vi "SV FRF State Manager.vi"(0 "FRF State":T10 {"spectrum info"."x-axis units" items=["Time (s)"=0, "Frequency-CB (Hz)"=1, "Frequency-CPB (Hz)"=1248, "Frequency-Arbitrary (Hz)"=2357, "Quefrency (s)"=2, "Revolutions (rev)"=3, "Order"=4, "Speed (RPM)"=11, "Speed (rad/s)"=21, "Index"=65535]; "spectrum info"."weighting filter" items=["Linear", "A-weighting", "B-weighting", "C-weighting", "ITU-R 468-4", "Dolby", "CCITT", "C-message", "Wb", "Wc", "Wd", "We", "Wf", "Wh", "Wj", "Wk", "Wm", "AES17 20 kHz lowpass", "AES17 40 kHz lowpass", "AES17 20 kHz highpass", "AES17 40 kHz highpass"]; "spectrum info"."dB reference [EU]" format="%.2f"; "spectrum info"."engineering units" items=["custom..."=0, "V"=1, "A"=21, "C"=30, "pC"=31, "s"=32, "-"=29, "Pa"=2, "N"=20, "g"=3, "m/s^2"=4, "m/s"=5, "m"=6, "mm/s"=12, "mm"=13, "micron/s"=14, "micron"=15, "in/s^2"=7, "in/s"=8, "in"=9, "mil/s"=10, "mil"=11, "rad/s^2"=16, "rad/s"=17, "rad"=18, "deg/s^2"=26, "deg/s"=27, "deg"=28, "RPM"=22, "cycle/s^2"=23, "Hz"=24, "cycle"=25, "strain"=19]; "spectrum info"."spectral info"."window" items=["None "=0, "Hanning"=1, "Hamming"=2, "Blackman-Harris"=3, "Exact Blackman"=4, "Blackman"=5, "Flat Top"=6, "4 Term B-Harris "=7, "7 Term B-Harris"=8, "Low Sidelobe"=9, "Force - Exponential"=10, "Gaussian"=62]; "Data"."coherence"."coherence" format="%.2f"; "Data"."coherence"."df" format="%.2f"; "Data"."coherence"."f0" format="%.2f"; "Data"."phase"."phase" format="%.2f"; "Data"."phase"."df" format="%.2f"; "Data"."phase"."f0" format="%.2f"; "Data"."magnitude"."magnitude" format="%.2p"; "Data"."magnitude"."df" format="%.2p"; "Data"."magnitude"."f0" format="%.2p"; "IDentifiers"."response node"."active node" format="%04.0f"; "IDentifiers"."reference node"."active node" format="%04.0f"}, 2 "Node IDentifiers":T8={"reference node"={"active node"=0, "coordinate"="+Y"}, "response node"={"active node"=0, "coordinate"="+Y"}} {"response node"."active node" format="%04.0f"; "reference node"."active node" format="%04.0f"}, 3 "FRF to add":T9 {"coherence"."coherence" format="%.2f"; "coherence"."df" format="%.2f"; "coherence"."f0" format="%.2f"; "phase"."phase" format="%.2f"; "phase"."df" format="%.2f"; "phase"."f0" format="%.2f"; "magnitude"."magnitude" format="%.2p"; "magnitude"."df" format="%.2p"; "magnitude"."f0" format="%.2p"}, 4 "spectrum info":T1={"channel name"="", "description"="", "x-axis units"=0, "spectral info"={"spectrum type"=enum."Power [Magnitude^2]", "linear/dB"=enum."linear", "window"=0, "window size"=0, "FFT size"=0}, "engineering units"=0, "custom label"="", "dB reference [EU]"=0.0, "peak units"=enum."rms", "weighting filter"=0, "spectral density?"=FALSE, "unit label"="", "spectrum skewed?"=FALSE, "complimentary spectrum units"=enum."none"} {"x-axis units" items=["Time (s)"=0, "Frequency-CB (Hz)"=1, "Frequency-CPB (Hz)"=1248, "Frequency-Arbitrary (Hz)"=2357, "Quefrency (s)"=2, "Revolutions (rev)"=3, "Order"=4, "Speed (RPM)"=11, "Speed (rad/s)"=21, "Index"=65535]; "weighting filter" items=["Linear", "A-weighting", "B-weighting", "C-weighting", "ITU-R 468-4", "Dolby", "CCITT", "C-message", "Wb", "Wc", "Wd", "We", "Wf", "Wh", "Wj", "Wk", "Wm", "AES17 20 kHz lowpass", "AES17 40 kHz lowpass", "AES17 20 kHz highpass", "AES17 40 kHz highpass"]; "dB reference [EU]" format="%.2f"; "engineering units" items=["custom..."=0, "V"=1, "A"=21, "C"=30, "pC"=31, "s"=32, "-"=29, "Pa"=2, "N"=20, "g"=3, "m/s^2"=4, "m/s"=5, "m"=6, "mm/s"=12, "mm"=13, "micron/s"=14, "micron"=15, "in/s^2"=7, "in/s"=8, "in"=9, "mil/s"=10, "mil"=11, "rad/s^2"=16, "rad/s"=17, "rad"=18, "deg/s^2"=26, "deg/s"=27, "deg"=28, "RPM"=22, "cycle/s^2"=23, "Hz"=24, "cycle"=25, "strain"=19]; "spectral info"."window" items=["None "=0, "Hanning"=1, "Hamming"=2, "Blackman-Harris"=3, "Exact Blackman"=4, "Blackman"=5, "Flat Top"=6, "4 Term B-Harris "=7, "7 Term B-Harris"=8, "Low Sidelobe"=9, "Force - Exponential"=10, "Gaussian"=62]}, 6 "action":u16(ring)=3 items=["Initialize to Empty", "Update State", "Delete from State", "Get Identifiers", "Get State"]) -> (12 "state changed":bool, 14 "FRF State out":T10 {"spectrum info"."x-axis units" items=["Time (s)"=0, "Frequency-CB (Hz)"=1, "Frequency-CPB (Hz)"=1248, "Frequency-Arbitrary (Hz)"=2357, "Quefrency (s)"=2, "Revolutions (rev)"=3, "Order"=4, "Speed (RPM)"=11, "Speed (rad/s)"=21, "Index"=65535]; "spectrum info"."weighting filter" items=["Linear", "A-weighting", "B-weighting", "C-weighting", "ITU-R 468-4", "Dolby", "CCITT", "C-message", "Wb", "Wc", "Wd", "We", "Wf", "Wh", "Wj", "Wk", "Wm", "AES17 20 kHz lowpass", "AES17 40 kHz lowpass", "AES17 20 kHz highpass", "AES17 40 kHz highpass"]; "spectrum info"."dB reference [EU]" format="%.2f"; "spectrum info"."engineering units" items=["custom..."=0, "V"=1, "A"=21, "C"=30, "pC"=31, "s"=32, "-"=29, "Pa"=2, "N"=20, "g"=3, "m/s^2"=4, "m/s"=5, "m"=6, "mm/s"=12, "mm"=13, "micron/s"=14, "micron"=15, "in/s^2"=7, "in/s"=8, "in"=9, "mil/s"=10, "mil"=11, "rad/s^2"=16, "rad/s"=17, "rad"=18, "deg/s^2"=26, "deg/s"=27, "deg"=28, "RPM"=22, "cycle/s^2"=23, "Hz"=24, "cycle"=25, "strain"=19]; "spectrum info"."spectral info"."window" items=["None "=0, "Hanning"=1, "Hamming"=2, "Blackman-Harris"=3, "Exact Blackman"=4, "Blackman"=5, "Flat Top"=6, "4 Term B-Harris "=7, "7 Term B-Harris"=8, "Low Sidelobe"=9, "Force - Exponential"=10, "Gaussian"=62]; "Data"."coherence"."coherence" format="%.2f"; "Data"."coherence"."df" format="%.2f"; "Data"."coherence"."f0" format="%.2f"; "Data"."phase"."phase" format="%.2f"; "Data"."phase"."df" format="%.2f"; "Data"."phase"."f0" format="%.2f"; "Data"."magnitude"."magnitude" format="%.2p"; "Data"."magnitude"."df" format="%.2p"; "Data"."magnitude"."f0" format="%.2p"; "IDentifiers"."response node"."active node" format="%04.0f"; "IDentifiers"."reference node"."active node" format="%04.0f"}, 16 "IDentifiers":T7(array[cluster]) {"response node"."active node" format="%04.0f"; "reference node"."active node" format="%04.0f"}, 17 "FRF requested":T9 {"coherence"."coherence" format="%.2f"; "coherence"."df" format="%.2f"; "coherence"."f0" format="%.2f"; "phase"."phase" format="%.2f"; "phase"."df" format="%.2f"; "phase"."f0" format="%.2f"; "magnitude"."magnitude" format="%.2p"; "magnitude"."df" format="%.2p"; "magnitude"."f0" format="%.2p"}, 18 "spectrum info":T1={"channel name"="", "description"="", "x-axis units"=0, "spectral info"={"spectrum type"=enum."Power [Magnitude^2]", "linear/dB"=enum."linear", "window"=0, "window size"=0, "FFT size"=0}, "engineering units"=0, "custom label"="", "dB reference [EU]"=0.0, "peak units"=enum."rms", "weighting filter"=0, "spectral density?"=FALSE, "unit label"="", "spectrum skewed?"=FALSE, "complimentary spectrum units"=enum."none"} {"x-axis units" items=["Time (s)"=0, "Frequency-CB (Hz)"=1, "Frequency-CPB (Hz)"=1248, "Frequency-Arbitrary (Hz)"=2357, "Quefrency (s)"=2, "Revolutions (rev)"=3, "Order"=4, "Speed (RPM)"=11, "Speed (rad/s)"=21, "Index"=65535]; "weighting filter" items=["Linear", "A-weighting", "B-weighting", "C-weighting", "ITU-R 468-4", "Dolby", "CCITT", "C-message", "Wb", "Wc", "Wd", "We", "Wf", "Wh", "Wj", "Wk", "Wm", "AES17 20 kHz lowpass", "AES17 40 kHz lowpass", "AES17 20 kHz highpass", "AES17 40 kHz highpass"]; "dB reference [EU]" format="%.2f"; "engineering units" items=["custom..."=0, "V"=1, "A"=21, "C"=30, "pC"=31, "s"=32, "-"=29, "Pa"=2, "N"=20, "g"=3, "m/s^2"=4, "m/s"=5, "m"=6, "mm/s"=12, "mm"=13, "micron/s"=14, "micron"=15, "in/s^2"=7, "in/s"=8, "in"=9, "mil/s"=10, "mil"=11, "rad/s^2"=16, "rad/s"=17, "rad"=18, "deg/s^2"=26, "deg/s"=27, "deg"=28, "RPM"=22, "cycle/s^2"=23, "Hz"=24, "cycle"=25, "strain"=19]; "spectral info"."window" items=["None "=0, "Hanning"=1, "Hamming"=2, "Blackman-Harris"=3, "Exact Blackman"=4, "Blackman"=5, "Flat Top"=6, "4 Term B-Harris "=7, "7 Term B-Harris"=8, "Low Sidelobe"=9, "Force - Exponential"=10, "Gaussian"=62]})   [LabVIEW 2017]
uses:
  <vilib>/addons/_NISVFA/_Shared subVIs/Controls/svc_Spectrum Info.ctl
  <vilib>/addons/_NISVFA/_Shared subVIs/Controls/svc_X-Axis Units.ctl
  <vilib>/addons/_NISVFA/_Shared subVIs/Controls/svc_Spectrum Type.ctl
  <vilib>/addons/_NISVFA/_Shared subVIs/Controls/svc_Engineering Units Text Ring.ctl
  <vilib>/addons/_NISVFA/_Shared subVIs/Controls/svc_Weighting Filter Text Ring.ctl
  <vilib>/addons/_NISVFA/_Shared subVIs/Controls/svc_Complimentary Spectrum Units.ctl
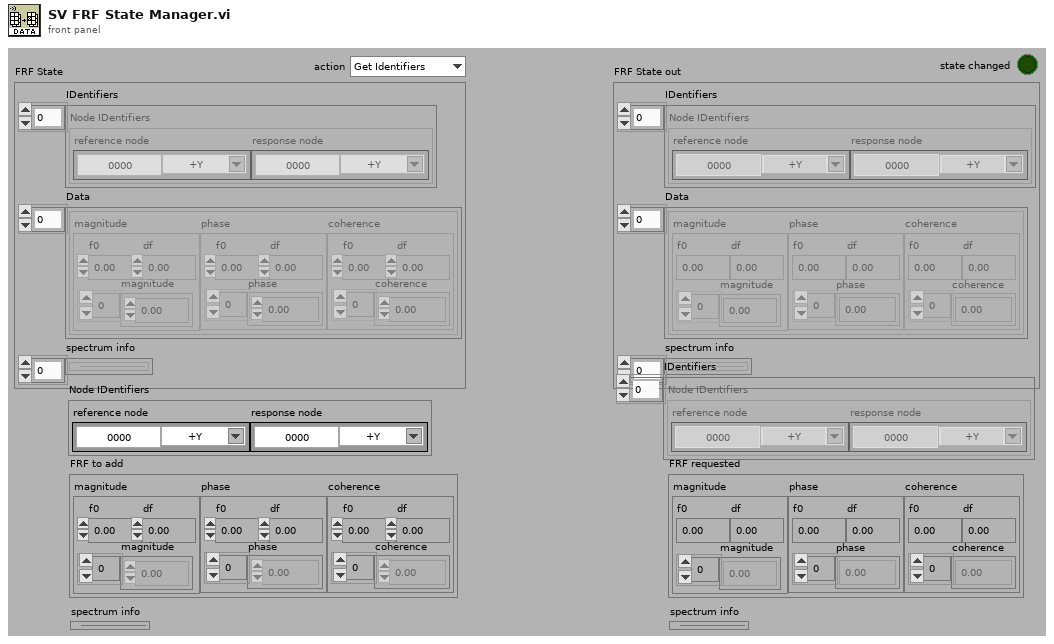
[diagram p1: front panel]
types:
  T1 = typedef "svc_Spectrum Info.ctl" = cluster{"channel name":string, "description":string, "x-axis units":T2, "spectral info":cluster{"spectrum type":T3, "linear/dB":enum16{"linear", "dB"}, "window":u16, "window size":i32, "FFT size":i32}, "engineering units":T4, "custom label":string, "dB reference [EU]":dbl, "peak units":enum16{"rms", "peak", "peak-peak"}, "weighting filter":T5, "spectral density?":bool, "unit label":string, "spectrum skewed?":bool, "complimentary spectrum units":T6}
  T2 = typedef "svc_X-Axis Units.ctl" = u16
  T3 = typedef "svc_Spectrum Type.ctl" = enum16{"FFT Spectrum [complex]", "Amplitude [Magnitude]", "Power [Magnitude^2]", "Cross Spectrum [complex]", "Frequency Response [Complex]"}
  T4 = typedef "svc_Engineering Units Text Ring.ctl" = u16
  T5 = typedef "svc_Weighting Filter Text Ring.ctl" = u16
  T6 = typedef "svc_Complimentary Spectrum Units.ctl" = enum16{"none", "radians", "degrees", "cycles", "imaginary"}
  T7 = cluster{"reference node":cluster{"active node":i32, "coordinate":string}, "response node":cluster{"active node":i32, "coordinate":string}}[]
  T8 = cluster{"reference node":cluster{"active node":i32, "coordinate":string}, "response node":cluster{"active node":i32, "coordinate":string}}
  T9 = cluster{"magnitude":cluster{"f0":dbl, "df":dbl, "magnitude":dbl[]}, "phase":cluster{"f0":dbl, "df":dbl, "phase":dbl[]}, "coherence":cluster{"f0":dbl, "df":dbl, "coherence":dbl[]}}
  T10 = cluster{"IDentifiers":cluster{"reference node":cluster{"active node":i32, "coordinate":string}, "response node":cluster{"active node":i32, "coordinate":string}}[], "Data":cluster{"magnitude":cluster{"f0":dbl, "df":dbl, "magnitude":dbl[]}, "phase":cluster{"f0":dbl, "df":dbl, "phase":dbl[]}, "coherence":cluster{"f0":dbl, "df":dbl, "coherence":dbl[]}}[], "spectrum info":T1[]}
  T11 = cluster{"magnitude":cluster{"f0":dbl, "df":dbl, "magnitude":dbl[]}, "phase":cluster{"f0":dbl, "df":dbl, "phase":dbl[]}, "coherence":cluster{"f0":dbl, "df":dbl, "coherence":dbl[]}}[]
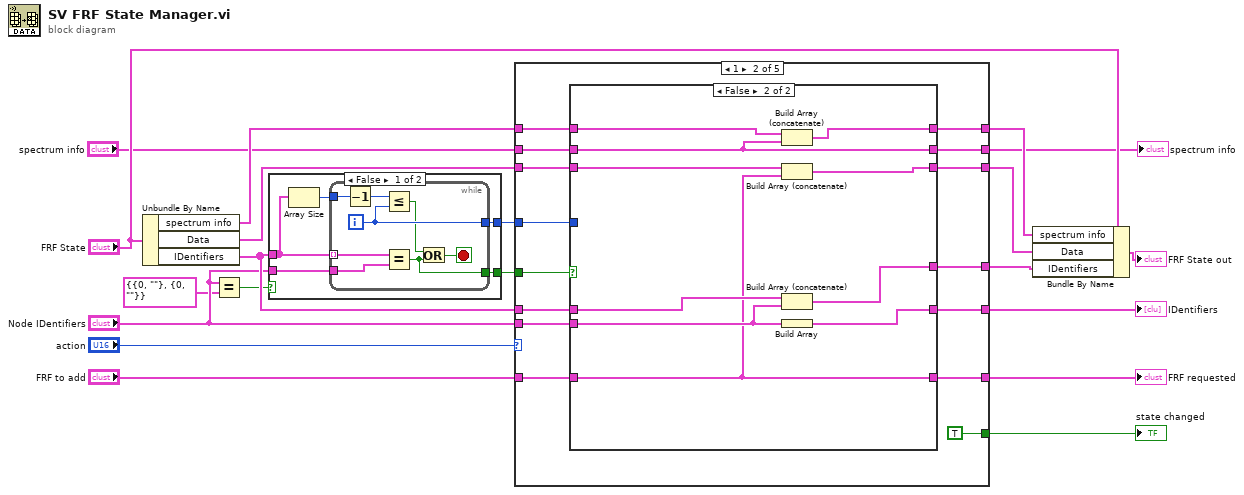
[diagram p0: block diagram]
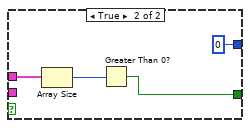
[diagram p2: hidden frame]
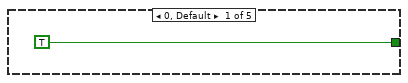
[diagram p3: hidden frame]
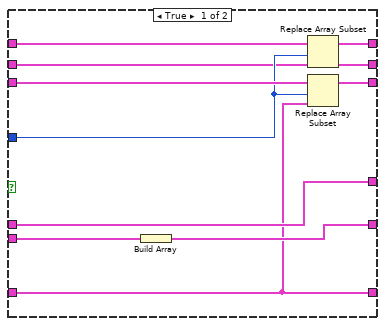
[diagram p4: hidden frame]
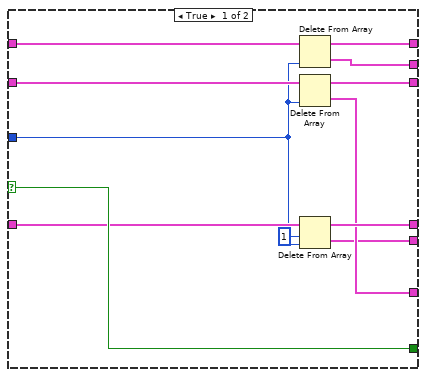
[diagram p6: hidden frame]
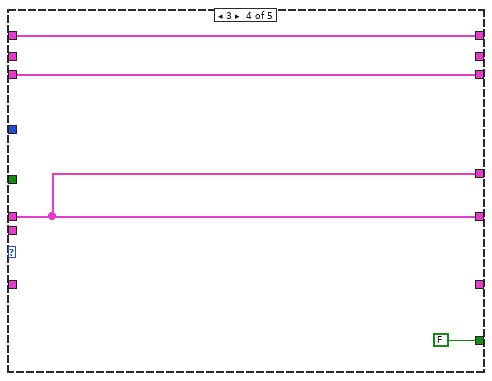
[diagram p7: hidden frame]
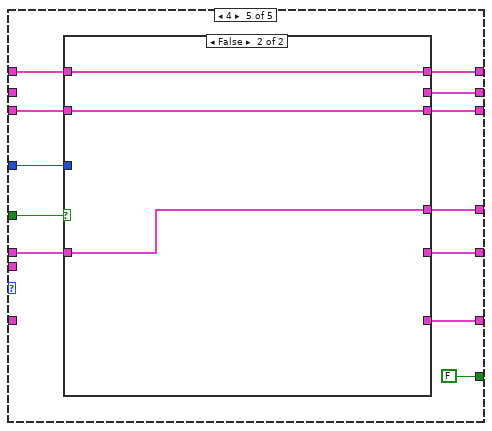
[diagram p8: hidden frame]
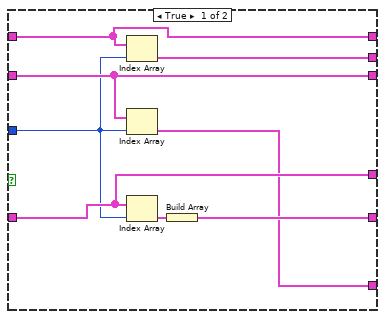
[diagram p9: hidden frame]
diagram:
  n1 = Unbundle By Name("FRF State") -> ("spectrum info"=w5:T1[], "Data"=w15:T11, "IDentifiers"=w12:T7)
  n2 = Equal?(x="Node IDentifiers", y=T8 {"reference node"={"active node"=0, "coordinate"=""}, "response node"={"active node"=0, "coordinate"=""}}) -> (x = y?=w11:bool)
  n3 = case shown="False" w11 {
    tunnel: [w24 0] -> w16
    tunnel: w12 -> [w23 w36]
    tunnel: [w22 w34] -> w7
    tunnel: "Node IDentifiers" -> [w21 _]
    frame False {
      n4 = Array Size(array=w23) -> (size(s)=w25:i32)
      n5 = while {
        tunnel: w23 -> [w26] mode=indexing
        tunnel: w21 -> [w33]
        tunnel: w25 -> [w31]
        tunnel: [w29] -> w24
        tunnel: [w27] -> w22
        i -> [w29]
        stop <- w30 stop-if-true
        n6 = Decrement(x=w31) -> (x-1=w32:i32)
        n7 = Less Or Equal?(x=w32, y=w29) -> (x <= y?=w28:bool)
        n8 = Equal?(x=w26, y=w33) -> (x = y?=w27:bool)
        n9 = Or(x=w28, y=w27) -> (x .or. y?=w30:bool)
      }
    }
    frame True {
      n10 = Array Size(array=w36) -> (size(s)=w35:i32)
      n11 = Greater Than 0?(x=w35) -> (x > 0?=w34:bool)
    }
  }
  n12 = case shown="1" "action" {
    tunnel: "Node IDentifiers" -> [_ w53 _ _ _]
    tunnel: "FRF to add" -> [_ w52 _ _ _]
    tunnel: [_ w44 w77 w104 w117] -> w18
    tunnel: [_ w51 w78 _ w116] -> w17
    tunnel: w16 -> [_ w48 w84 _ w115]
    tunnel: w15 -> [_ w50 w85 w105 w114]
    tunnel: [_ w47 w83 w105 w113] -> w13
    tunnel: w12 -> [_ w49 w80 w104 w112]
    tunnel: [_ w45 w79 w104 w111] -> w10
    tunnel: w7 -> [_ w46 w82 _ w110]
    tunnel: [TRUE TRUE w81 FALSE FALSE] -> w6
    tunnel: w5 -> [_ w42 w76 w102 w108]
    tunnel: [_ w41 w75 w102 w107] -> w4
    tunnel: "spectrum info" -> [_ w40 _ _ _]
    tunnel: [_ w39 w74 _ w106] -> w2
    frame 0, Default {
    }
    frame 1 {
      n13 = case shown="False" w46 {
        tunnel: w50 -> [w63 w73]
        tunnel: w48 -> [w56 _]
        tunnel: w52 -> [w59 w67]
        tunnel: w49 -> [w61 w72]
        tunnel: w53 -> [w58 w68]
        tunnel: [w62 w71] -> w47
        tunnel: [w61 w70] -> w45
        tunnel: [w59 w67] -> w51
        tunnel: [w60 w69] -> w44
        tunnel: w42 -> [w57 w66]
        tunnel: [w55 w65] -> w41
        tunnel: w40 -> [w54 w64]
        tunnel: [w54 w64] -> w39
        frame True {
          n14 = Build Array(w58) -> (w60:T7)
          n15 = Replace Array Subset(array=w57, new element=w54, index=w56) -> (w55:T1[])
          n16 = Replace Array Subset(array=w63, new element=w59, index=w56) -> (w62:T11)
        }
        frame False {
          n17 = Build Array (concatenate)(w66, w64) -> (w65:T1[])
          n18 = Build Array (concatenate)(w73, w67) -> (w71:T11)
          n19 = Build Array (concatenate)(w72, w68) -> (w70:T7)
          n20 = Build Array(w68) -> (w69:T7)
        }
      }
    }
    frame 2 {
      n21 = case shown="False" w82 {
        selector: w82 -> [w97 w100]
        tunnel: w85 -> [w96 w101]
        tunnel: w84 -> [w88 _]
        tunnel: w80 -> [w94 w99]
        tunnel: [w95 w101] -> w83
        tunnel: [w93 w99] -> w79
        tunnel: [w97 w100] -> w81
        tunnel: [w92 _] -> w78
        tunnel: [w91 _] -> w77
        tunnel: [w86 w98] -> w75
        tunnel: w76 -> [w89 w98]
        tunnel: [w87 _] -> w74
        frame True {
          n22 = Delete From Array(array=w89, index=w88) -> (deleted portion=w87:T1, array with subset deleted=w86:T1[])  [unwired: 1 in]
          n23 = Delete From Array(array=w96, index=w88) -> (deleted portion=w92:T9, array with subset deleted=w95:T11)  [unwired: 1 in]
          n24 = Delete From Array(array=w94, length=1, index=w88) -> (deleted portion=w91:T7, array with subset deleted=w93:T7)
        }
        frame False {
        }
      }
    }
    frame 3 {
    }
    frame 4 {
      n25 = case shown="False" w110 {
        tunnel: w114 -> [w125 w128]
        tunnel: w115 -> [w120 _]
        tunnel: w112 -> [w122 w127]
        tunnel: [w125 w128] -> w113
        tunnel: [w123 _] -> w117
        tunnel: [w121 _] -> w116
        tunnel: [w122 w127] -> w111
        tunnel: w108 -> [w118 w126]
        tunnel: [w118 w126] -> w107
        tunnel: [w119 _] -> w106
        frame True {
          n26 = Index Array(array=w118, index=w120) -> (element=w119:T1)
          n27 = Index Array(array=w125, index=w120) -> (element=w121:T9)
          n28 = Index Array(array=w122, index=w120) -> (element=w124:T8)
          n29 = Build Array(w124) -> (w123:T7)
        }
        frame False {
        }
      }
    }
  }
  "FRF requested" <- w17
  "IDentifiers" <- w18
  "state changed" <- w6
  "spectrum info" <- w2
  n30 = Bundle By Name(cluster="FRF State", "spectrum info"=w4, "Data"=w13, "IDentifiers"=w10) -> (→"FRF State out":T10)
